vi "FPGA_Main.vi"() -> ()   [LabVIEW 2024]
uses:
  LED_Status.ctl
  <vilib>/rvi/Emulation/niFpgaGetClockAttributes.vi
  <vilib>/rvi/Emulation/niFpgaSctlEmulationGetInTimedLoop.vi
  <vilib>/rvi/Emulation/niFpgaEmulationReportErrorSimple.vi
  <vilib>/rvi/eio/common/nirviEmuTemplateMethod_errors.vi
  <vilib>/rvi/Emulation/niFpgaCriticalErrorInLSC.vi
  <vilib>/eio/EIONode/EIONode.xnode
panel:
  in  "Count(mSec)":u32
  out "Numeric":i32
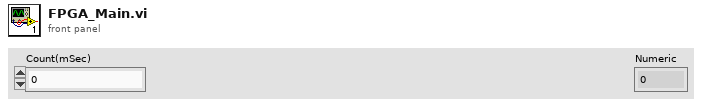
[diagram p1: front panel]
types:
  T1 = typedef "LED_Status.ctl" = enum8{"LED_1", "LED_2", "LED_3"}
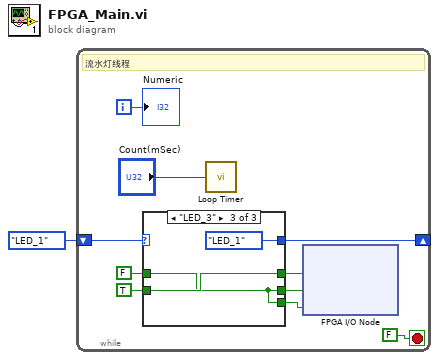
[diagram p0: block diagram]
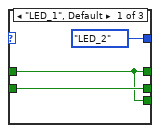
[diagram p2: hidden frame]
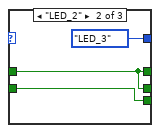
[diagram p3: hidden frame]
diagram:
  n1 = while {
    shift-right: [w9] -> _
    shift-left: LED_Status."LED_1" -> [w10]
    i -> [w2]
    stop <- FALSE stop-if-true
    # "流水灯线程"
    n2 = case shown="\"LED_3\"" w10 {
      tunnel: [LED_Status."LED_2" LED_Status."LED_3" LED_Status."LED_1"] -> w9
      tunnel: TRUE -> [w13 w16 w19]
      tunnel: FALSE -> [w12 w15 w18]
      tunnel: [w12 w15 w19] -> w5
      tunnel: [w13 w15 w18] -> w4
      tunnel: [w12 w16 w18] -> w3
      frame "LED_1", Default {
      }
      frame "LED_2" {
      }
      frame "LED_3" {
      }
    }
    n3 = call "Loop Timer"("Count(mSec)"="Count(mSec)") -> ()  [unwired: 1 out]
    n4 = xnode "FPGA I/O Node"("User LED1"=w5, "User LED2"=w4, "User LED3"=w3) -> ()  [unwired: 3 in, 3 out]
    "Numeric" <- w2
  }
